vi "Band Magnitude - Peak (CPM).vi"(0 "power spectrum [EU^2 rms]":cluster{"f0":dbl, "df":dbl, "magnitude":sgl[]}, 5 "Start":dbl, 7 "Stop":dbl=60000.0, 11 "error in (no error)":errorcluster) -> (6 "Max Peak In Band [EU rms]":sgl=nan format="%.2f", 15 "error out":errorcluster)   [LabVIEW 2017, in "VibrationAnalysisFunctions.lvlib"]
uses:
  <vilib>/addons/InsightCM/Utilities/Analysis/Vibration/VibrationAnalysisFunctions.lvlib
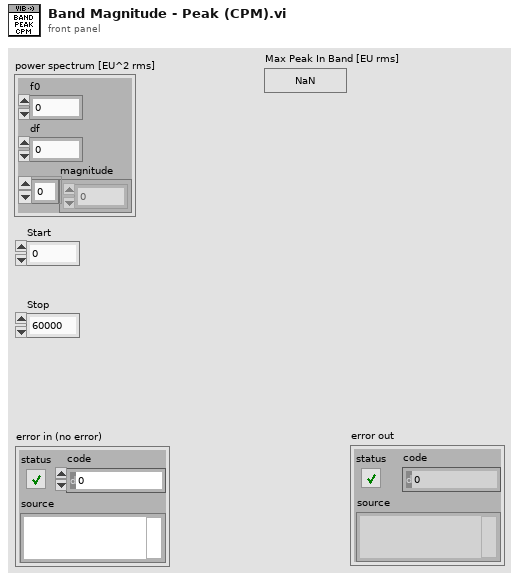
[diagram p1: front panel]
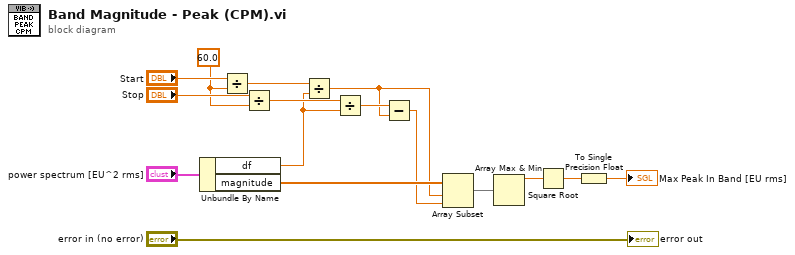
[diagram p0: block diagram]
diagram:
  w13 = 60.0 ("y")
  n1 = Unbundle By Name("power spectrum [EU^2 rms]") -> ("df"=w8:dbl, "magnitude"=w6:sgl[])
  n2 = Divide(x="Start", y=w13) -> (x/y=w10:dbl)
  n3 = Divide(x="Stop", y=w13) -> (x/y=w9:dbl)
  n4 = Divide(x=w10, y=w8) -> (x/y=w5:dbl)
  n5 = Divide(x=w9, y=w8) -> (x/y=w7:dbl)
  n6 = Subtract(x=w7, y=w5) -> (x-y=w4:dbl)
  n7 = Array Subset(array=w6, index=w5, length=w4) -> (w3:sgl[])
  n8 = Array Max & Min(array=w3) -> (max value=w2:sgl)  [unwired: 3 out]
  n9 = Square Root(x=w2) -> (sqrt(x)=w1:sgl)
  n10 = To Single Precision Float(number=w1) -> (single precision float=→"Max Peak In Band [EU rms]":sgl)
  "error out" <- "error in (no error)"
